vi "Daemon_CreateStore Launcher.vi"(7 "Dialog Name":string, 8 "error in":errorcluster, 9 "Daemon Name (\"\": use VI name)":string, 10 "Dialog Text":string, 11 "jModule":refnum<class "jModule.lvclass">) -> (0 "error out":errorcluster, 1 "Daemon Name":string, 2 "VI Refnum":refnum<vi>, 3 "jModule":refnum<class "jModule.lvclass">)   [LabVIEW 2020]
doc: "This VI is used to launch a Daemon that prompts the user to make a choice.\n\n<b> IMPORTANT:</b> You should wire the jModule output from this Launcher. The Launcher adds the Daemon to the jModule so that jModule can abort the deamon in the event of a software shutdown.\n\n<b>NOTE:</b> Daemons send jMsgs only to their callers; their callers need not subscribe to receive their Daemons' jMsgs\ncreated using\nJSMA Daemon Template - Two Button Prompt 0.2.0.2\nRob Humfeld - Jet Engineering\nCopyright (c) 2020, Jet Engineering"
uses:
  <userlib>/JET Engineering/JSMA/Libraries/jModule Class/jModule.lvclass
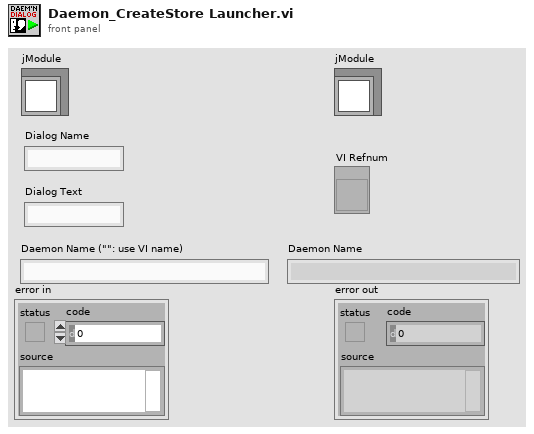
[diagram p1: front panel]
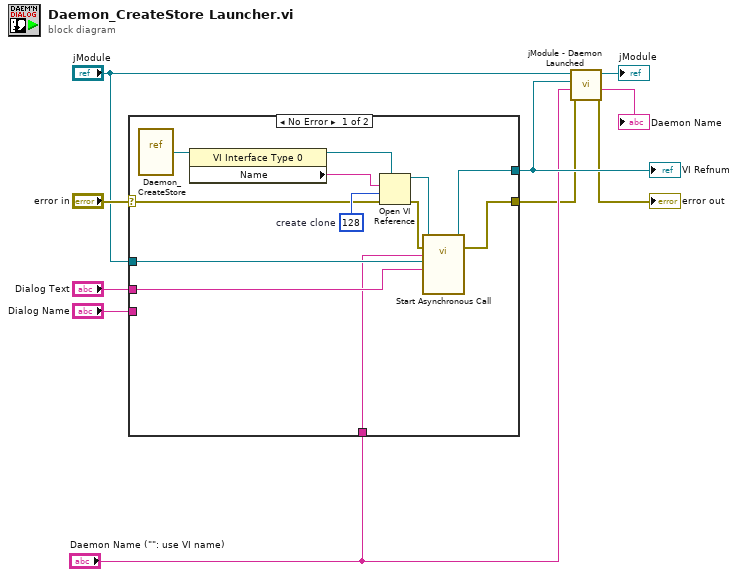
[diagram p0: block diagram]
diagram:
  n1 = case shown="No Error" "error in" {
    selector: "error in" -> [w13 w23]
    tunnel: "jModule" -> [w22 _]
    tunnel: [w20 w23] -> w4
    tunnel: [w14 _] -> w6
    tunnel: "Dialog Name" -> [_ _]
    tunnel: "Dialog Text" -> [w12 _]
    tunnel: "Daemon Name (\"\": use VI name)" -> [w11 _]
    frame No Error {
      w15 = 128  # create clone
      n2 = vi-ref "Daemon_CreateStore.vi"() -> (w19:refnum<vi>)
      n3 = property class="VI Interface Type 0"(reference=w19) -> (reference out=w18:refnum<vi>, "Name"=w16:string)  [unwired: 1 in, 1 out]
      n4 = Open VI Reference(type specifier VI Refnum (for type only)=w18, vi path=w16, options=w15, error in (no error)=w13) -> (vi reference=w17:refnum<vi>, error out=w21:errorcluster)  [unwired: 2 in]
      n5 = call-by-ref "Start Asynchronous Call"(reference=w17, error in=w21, "Dialog Name"=w11, "Dialog Parameters"=w12, "jModule"=w22) -> (reference out=w14:refnum<vi>, error out=w20:errorcluster)  [unwired: 9 in]
    }
    frame Error {
    }
  }
  "VI Refnum" <- w6
  n6 = call <userlib>:"jModule - Daemon Launched.vi"("error in (no error)"=w4, "Daemon Name (\"\": use VI name)"="Daemon Name (\"\": use VI name)", "vi reference"=w6, "jModule"="jModule") -> ("error out"=→"error out":errorcluster, "Daemon Name"=→"Daemon Name":string, "jModule"=→"jModule":refnum<class "jModule.lvclass">)  [unwired: 5 in]
